vi "Day 3 - RE Python.vi"() -> ()   [LabVIEW 2019]
uses:
  981daa9d-93ea-4baa-a2ea-66ed7e93d154.vi
panel:
  out "Split String":string[][](array[string])
  in  "Error In":errorcluster
  in  "Relative Path to Input File":string
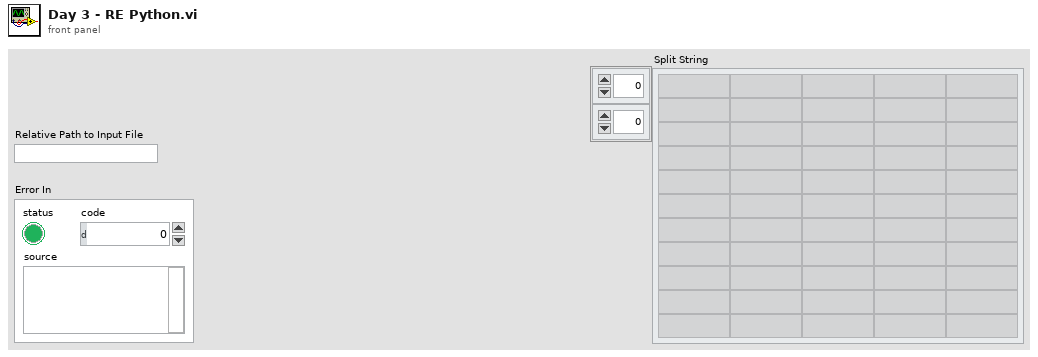
[diagram p1: front panel]
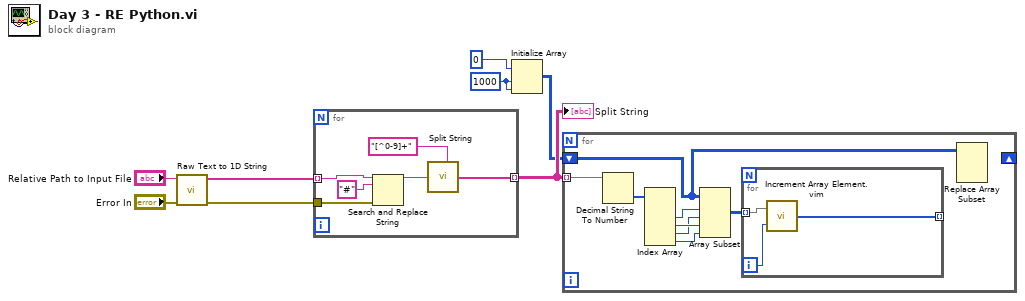
[diagram p0: block diagram]
diagram:
  w3 = 1000 ("dimension size")
  n1 = call "Raw Text to 1D String.vi"("Error In"="Error In", "Relative Path to Input File"="Relative Path to Input File") -> ("Error Out"=w5:errorcluster, "1D String Array"=w6:string[])  [unwired: 8 in]
  n2 = for {
    tunnel: w6 -> [w11] mode=indexing
    tunnel: w5 -> [w10]
    tunnel: [w9] -> w2 mode=indexing
    n3 = Search and Replace String(input string=w11, search string="#", error in=w10) -> (result string=w12:string)  [unwired: 5 in, 3 out]
    n4 = call <vilib>:"Split String.vi"("Split Pattern"="[^0-9]+", "Input String"=w12) -> ("Split String"=w9:string[])  [unwired: 5 in]
  }
  "Split String" <- w2
  n5 = Initialize Array(0 ("element"), w3, w3) -> (w1:i32[][])
  n6 = for {
    tunnel: w2 -> [w22] mode=indexing
    shift-right: _ -> [_]
    shift-left: w1 -> [w15]
    n7 = Decimal String To Number(string=w22) -> (number=w21:i32[])  [unwired: 2 in, 1 out]
    n8 = Index Array(array=w21) -> (element #2=w20:i32, element #3=w19:i32, element #4=w18:i32, element #5=w17:i32)  [unwired: 5 in, 1 out]
    n9 = Array Subset(array=w15, index (row)=w20, length (row)=w18, index (col)=w19, length (col)=w17) -> (w16:i32[][])
    n10 = for {
      tunnel: w16 -> [w25] mode=indexing
      tunnel: [w23] -> _ mode=indexing
      i -> [w24]
      n11 = call "Increment Array Element.vim"("index"=w24, "array in"=w25) -> ("array out"=w23:i32[])
    }
    n12 = Replace Array Subset(array=w15) -> ()  [unwired: 3 in, 1 out]
  }
